vi "BonOMM-SAOMM.Test.vi"() -> ()   [LabVIEW 2011] (continued)
          n234 = property on="Offset OK" class="Bool (strict)"("DisabledEnum"=w454) -> ()  [unwired: 2 in, 2 out]
          n235 = local write "PixScale1"(w356) -> ()
          n236 = To Unsigned Word Integer(number=w325) -> (unsigned 16bit integer=w327:u16)
          n237 = To Unsigned Word Integer(number=w324) -> (unsigned 16bit integer=w326:u16)
          n238 = call-poly <vilib>:"Read Key.vi"("section"=w260, "error in (no error)"=w372, "key"="pixscale2", "refnum"=w367) -> ("error out"=w363:errorcluster, "value"=w355:dbl, "refnum out"=w364:T24)  [unwired: 4 in, 1 out]
          n239 = local write "Naxis2"(w327) -> ()
          n240 = local write "Naxis1"(w326) -> ()
          n241 = local write "PixScale2"(w355) -> ()
          n242 = property on="TableXYPos" class="XYGraph (strict)"("Active Cursor"=u32 0) -> (error out=w523:errorcluster)  [unwired: 2 in, 1 out]
          n243 = call-poly <vilib>:"Read Key.vi"("section"=w260, "error in (no error)"=w363, "key"="ROIWidth", "refnum"=w364) -> ("error out"=w365:errorcluster, "value"=w321:u32, "refnum out"=w366:T24)  [unwired: 4 in, 1 out]
          n244 = property on="TableXYPos" class="XYGraph (strict)"("PlotImages.Back"=picture data[5B] ("Plot Images:Back")) -> ()  [unwired: 2 in, 2 out]
          n245 = call-poly <vilib>:"Read Key.vi"("section"=w260, "error in (no error)"=w365, "key"="ROIHeight", "refnum"=w366) -> ("error out"=w273:errorcluster, "value"=w322:u32, "refnum out"=w274:T24)  [unwired: 4 in, 1 out]
          n246 = property on="ImgArray" class="IntGraph (strict)"("X Scale.Scale Fit"=w531, "Y Scale.Scale Fit"=w531, "Z Scale.Scale Fit"=u8 2) -> ()  [unwired: 2 in, 2 out]
          n247 = property on="LVDT-RA-coarse" class="WFGraph (strict)"("YScale.Maximum"=20.0 ("Y Scale.Range:Maximum"), "YScale.Minimum"=-3.0 ("Y Scale.Range:Minimum")) -> ()  [unwired: 2 in, 2 out]
          n248 = property on="TableXYPos" class="XYGraph (strict)"(error in=w523, "Cursor.Cursor X"=w519, "Cursor.Cursor Y"=w519) -> (error out=w524:errorcluster)  [unwired: 1 in, 1 out]
          n249 = property on="LowSNR" class="Bool (strict)"("Visible"=w215, "Blinking"=w215) -> ()  [unwired: 2 in, 2 out]
          n250 = property on="Saturé" class="Bool (strict)"("Visible"=w215, "Blinking"=w215) -> ()  [unwired: 2 in, 2 out]
          n251 = call-poly <vilib>:"Read Key.vi"("section"=w260, "error in (no error)"=w273, "key"="DefaultROIOffset", "refnum"=w274) -> ("error out"=w265:errorcluster, "value"=w266:u32, "refnum out"=w264:T24)  [unwired: 4 in, 1 out]
          n252 = To Unsigned Word Integer(number=w322) -> (unsigned 16bit integer=w323:u16)
          n253 = To Unsigned Word Integer(number=w321) -> (unsigned 16bit integer=w320:u16)
          n254 = local write "ROIHeight"(w323) -> ()
          n255 = local write "ROIWidth"(w320) -> ()
          n256 = property on="TableXYPos" class="XYGraph (strict)"(error in=w524, "Active Cursor"=u32 1) -> (error out=w522:errorcluster)  [unwired: 1 in, 1 out]
          n257 = call-poly <vilib>:"Read Key.vi"("section"=w260, "error in (no error)"=w265, "key"="DefaultBinning", "refnum"=w264) -> ("error out"=w254:errorcluster, "value"=w267:u32, "refnum out"=w255:T24)  [unwired: 4 in, 1 out]
          n258 = call-poly <vilib>:"Read Key.vi"("section"=w249, "error in (no error)"=w254, "key"="GuideRateRA", "refnum"=w255) -> ("error out"=w340:errorcluster, "value"=w331:dbl, "refnum out"=w341:T24)  [unwired: 4 in, 1 out]
          n259 = local write "RateRA"(w331) -> ()
          n260 = call-poly <vilib>:"Read Key.vi"("section"=w249, "error in (no error)"=w340, "key"="GuideRateDEC", "refnum"=w341) -> ("error out"=w247:errorcluster, "value"=w330:dbl, "refnum out"=w248:T24)  [unwired: 4 in, 1 out]
          n261 = local write "RateDEC"(w330) -> ()
          n262 = call-poly <vilib>:"Read Key.vi"("section"=w249, "error in (no error)"=w247, "key"="HexXRate", "refnum"=w248) -> ("error out"=w253:errorcluster, "value"=w244:dbl, "refnum out"=w252:T24)  [unwired: 4 in, 1 out]
          n263 = local write "HexXRate"(w244) -> ()
          n264 = call-poly <vilib>:"Read Key.vi"("section"=w249, "error in (no error)"=w253, "key"="HexYRate", "refnum"=w252) -> ("error out"=w245:errorcluster, "value"=w243:dbl, "refnum out"=w246:T24)  [unwired: 4 in, 1 out]
          n265 = local write "HexYRate"(w243) -> ()
          n266 = call-poly <vilib>:"Read Key.vi"("section"=w249, "error in (no error)"=w245, "key"="BacklashRA", "refnum"=w246) -> ("error out"=w339:errorcluster, "value"=w329:dbl, "refnum out"=w342:T24)  [unwired: 4 in, 1 out]
          n267 = local write "BacklashRA"(w329) -> ()
          n268 = call-poly <vilib>:"Read Key.vi"("section"=w249, "error in (no error)"=w339, "key"="BacklashDEC", "refnum"=w342) -> ("error out"=w346:errorcluster, "value"=w328:dbl, "refnum out"=w345:T24)  [unwired: 4 in, 1 out]
          n269 = local write "BacklashDEC"(w328) -> ()
          n270 = call-poly <vilib>:"Read Key.vi"("section"=w249, "error in (no error)"=w346, "key"="GuiderAgg", "refnum"=w345) -> ("error out"=w344:errorcluster, "value"=w332:dbl, "refnum out"=w343:T24)  [unwired: 4 in, 1 out]
          n271 = local write "Corr%"(w332) -> ()
          n272 = call-poly <vilib>:"Read Key.vi"("section"=w249, "error in (no error)"=w344, "key"="GuiderTreshold", "refnum"=w343) -> ("error out"=w335:errorcluster, "value"=w333:dbl, "refnum out"=w336:T24)  [unwired: 4 in, 1 out]
          n273 = local write "CorrTreshold"(w333) -> ()
          n274 = call-poly <vilib>:"Read Key.vi"("section"=w249, "error in (no error)"=w335, "key"="SNRTreshold", "refnum"=w336) -> ("error out"=w256:errorcluster, "value"=→"SNRtreshold":dbl, "refnum out"=w257:T24)  [unwired: 4 in, 1 out]
          n275 = call-poly <vilib>:"Read Key.vi"("section"=w258, "error in (no error)"=w256, "key"="UAxisOffset", "refnum"=w257) -> ("error out"=w281:errorcluster, "value"=w276:dbl, "refnum out"=w282:T24)  [unwired: 4 in, 1 out]
          n276 = local write "DefaultUAxisOffset"(w276) -> ()
          n277 = call-poly <vilib>:"Read Key.vi"("section"=w258, "error in (no error)"=w281, "key"="VAxisOffset", "refnum"=w282) -> ("error out"=w279:errorcluster, "value"=w275:dbl, "refnum out"=w280:T24)  [unwired: 4 in, 1 out]
          n278 = local write "DefaultVAxisOffset"(w275) -> ()
          n279 = call-poly <vilib>:"Read Key.vi"("section"=w258, "error in (no error)"=w279, "key"="Sampling", "refnum"=w280) -> ("error out"=w316:errorcluster, "value"=→"Sampling rate":i32, "refnum out"=w317:T24)  [unwired: 4 in, 1 out]
          n280 = call-poly <vilib>:"Read Key.vi"("section"=w258, "error in (no error)"=w316, "key"="DataLenght", "refnum"=w317) -> ("error out"=w238:errorcluster, "value"=w334:i32, "refnum out"=w237:T24)  [unwired: 4 in, 1 out]
          n281 = local write "ConsideredLenght"(w334) -> ()
          n282 = local write "Flat"(w473) -> ()
          n283 = call-poly <vilib>:"Read Key.vi"("section"=w207, "error in (no error)"=w238, "key"="PRAMMS-SG", "refnum"=w237) -> ("error out"=w213:errorcluster, "value"=w235:u32, "refnum out"=w214:T24)  [unwired: 4 in, 1 out]
          n284 = property on="TableXYPos" class="XYGraph (strict)"(error in=w522, "Cursor.Cursor X"=w518, "Cursor.Cursor Y"=w518) -> ()  [unwired: 1 in, 2 out]
          n285 = local write "Néon"(w473) -> ()
          n286 = local write "Signature"(w235) -> ()
          n287 = To Unsigned Word Integer(number=w267) -> (unsigned 16bit integer=w268:u16)
          n288 = To Unsigned Word Integer(number=w266) -> (unsigned 16bit integer=w270:u16)
          n289 = To Unsigned Word Integer(number=w266) -> (unsigned 16bit integer=w269:u16)
          n290 = local write "Arc"(w473) -> ()
          n291 = local write "Binning"(w268) -> ()
          n292 = local write "ROIYOffset"(w270) -> ()
          n293 = local write "ROIXOffset"(w269) -> ()
          n294 = local write "NeonOn"(w473) -> ()
          n295 = local write "ArcOn"(w473) -> ()
          n296 = global read "Globals.vi" "BonOMM VI Refnum"() -> (w283:refnum<vi>)
          n297 = call-poly <vilib>:"Read Key.vi"("section"=w207, "error in (no error)"=w213, "key"="tempspd", "refnum"=w214) -> ("error out"=w210:errorcluster, "value"=w204:u32, "refnum out"=w211:T24)  [unwired: 4 in, 1 out]
          n298 = local write "FlatOn"(w473) -> ()
          n299 = Initialize Array(0.0, 0) -> (w241:dbl[])
          n300 = Initialize Array(sgl 0.0, w516, w516) -> (w515:sgl[][])
          n301 = Bundle(w413, w413, w413) -> (w412:cluster{string, string, string})  [unwired: 1 in]
          n302 = local write "ImgData"(w515) -> ()
          n303 = local write "MC_connect"(FALSE) -> ()
          n304 = call-poly <vilib>:"Read Key.vi"("section"=w207, "error in (no error)"=w210, "key"="tempvrn", "refnum"=w211) -> ("error out"=w208:errorcluster, "value"=w205:string, "refnum out"=w209:T24)  [unwired: 4 in, 1 out]
          n305 = call-poly <vilib>:"Read Key.vi"("section"=w302, "error in (no error)"=w208, "key"="xgain", "refnum"=w209) -> ("error out"=w309:errorcluster, "value"=→"Gain X":dbl, "refnum out"=w308:T24)  [unwired: 4 in, 1 out]
          n306 = call-poly <vilib>:"Read Key.vi"("section"=w302, "error in (no error)"=w309, "key"="ygain", "refnum"=w308) -> ("error out"=w304:errorcluster, "value"=→"Gain Y":dbl, "refnum out"=w305:T24)  [unwired: 4 in, 1 out]
          n307 = call-poly <vilib>:"Read Key.vi"("section"=w302, "error in (no error)"=w304, "key"="zgain", "refnum"=w305) -> ("error out"=w314:errorcluster, "value"=→"Gain Z":dbl, "refnum out"=w313:T24)  [unwired: 4 in, 1 out]
          n308 = call-poly <vilib>:"Read Key.vi"("section"=w302, "error in (no error)"=w314, "key"="ugain", "refnum"=w313) -> ("error out"=w312:errorcluster, "value"=→"Gain U":dbl, "refnum out"=w311:T24)  [unwired: 4 in, 1 out]
          n309 = call-poly <vilib>:"Read Key.vi"("section"=w302, "error in (no error)"=w312, "key"="vgain", "refnum"=w311) -> ("error out"=w262:errorcluster, "value"=→"Gain V":dbl, "refnum out"=w263:T24)  [unwired: 4 in, 1 out]
          n310 = call-poly <vilib>:"Read Key.vi"("section"="options", "error in (no error)"=w262, "default value"=FALSE, "key"="autoconnect", "refnum"=w263) -> ("error out"=w378:errorcluster, "value"=w374:bool, "refnum out"=w379:T24)  [unwired: 3 in, 1 out]
          n311 = local write "AutoConnect?"(w374) -> ()
          n312 = call-poly <vilib>:"Read Key.vi"("section"=w382, "error in (no error)"=w378, "key"="secperpulse", "refnum"=w379) -> ("error out"=w392:errorcluster, "value"=w231:dbl, "refnum out"=w394:T24)  [unwired: 4 in, 1 out]
          "arcsec/pulse" <- w231
          n313 = call-poly <vilib>:"Read Key.vi"("section"=w382, "error in (no error)"=w392, "key"="naxis1", "refnum"=w394) -> ("error out"=w391:errorcluster, "value"=w232:dbl, "refnum out"=w393:T24)  [unwired: 4 in, 1 out]
          n314 = local write "NaxisMax"(w232) -> ()
          n315 = Multiply(x=w232, y=w231) -> (x*y=w230:dbl)
          n316 = call-poly <vilib>:"Read Key.vi"("section"=w382, "error in (no error)"=w391, "key"="represent", "refnum"=w393) -> ("error out"=w423:errorcluster, "value"=w420:dbl, "refnum out"=w424:T24)  [unwired: 4 in, 1 out]
          "Représentation" <- w420
          n317 = expression code="x/60"(w230) -> (→"RangeTable":dbl)
          n318 = call-poly <vilib>:"Read Key.vi"("section"=w382, "error in (no error)"=w423, "key"="cenx", "refnum"=w424) -> ("error out"=w505:errorcluster, "value"=w504:i32, "refnum out"=w506:T24)  [unwired: 4 in, 1 out]
          n319 = local write "CentreTel X"(w504) -> ()
          n320 = call-poly <vilib>:"Read Key.vi"("section"=w382, "error in (no error)"=w505, "key"="ceny", "refnum"=w506) -> ("error out"=w497:errorcluster, "value"=w503:i32, "refnum out"=w498:T24)  [unwired: 4 in, 1 out]
          n321 = local write "CentreTel Y"(w503) -> ()
          n322 = call-poly <vilib>:"Read Key.vi"("section"=w382, "error in (no error)"=w497, "key"="refx", "refnum"=w498) -> ("error out"=w502:errorcluster, "value"=w496:i32, "refnum out"=w501:T24)  [unwired: 4 in, 1 out]
          n323 = local write "Reference X"(w496) -> ()
          n324 = call-poly <vilib>:"Read Key.vi"("section"=w382, "error in (no error)"=w502, "key"="refy", "refnum"=w501) -> ("error out"=w433:errorcluster, "value"=w495:i32, "refnum out"=w434:T24)  [unwired: 4 in, 1 out]
          n325 = local write "Reference Y"(w495) -> ()
          n326 = Less Or Equal?(x=w420, y=70.0) -> (x <= y?=w418:bool)
          n327 = call-poly <vilib>:"Read Key.vi"("section"=w382, "error in (no error)"=w433, "key"="rangex", "refnum"=w434) -> ("error out"=w435:errorcluster, "value"=w438:i32, "refnum out"=w436:T24)  [unwired: 4 in, 1 out]
          n328 = local write "Rangement X"(w438) -> ()
          n329 = Select(t=T17."Enabled" ("Disabled"), s=w418, f=T17."Disabled" ("Disabled")) -> (s? t:f=w415:T17)
          n330 = call-poly <vilib>:"Read Key.vi"("section"=w382, "error in (no error)"=w435, "key"="rangey", "refnum"=w436) -> ("error out"=w429:errorcluster, "value"=w439:i32, "refnum out"=w430:T24)  [unwired: 4 in, 1 out]
          n331 = local write "Rangement Y"(w439) -> ()
          n332 = property on="GetDSS" class="Bool (strict)"("DisabledEnum"=w415) -> ()  [unwired: 2 in, 2 out]
          n333 = call-poly <vilib>:"Read Key.vi"("section"=w382, "error in (no error)"=w429, "key"="rangez", "refnum"=w430) -> ("error out"=w427:errorcluster, "value"=w426:i32, "refnum out"=w428:T24)  [unwired: 4 in, 1 out]
          n334 = local write "Rangement Z"(w426) -> ()
          n335 = call-poly <vilib>:"Read Key.vi"("section"=w382, "error in (no error)"=w427, "key"="vrapid", "refnum"=w428) -> ("error out"=w465:errorcluster, "value"=→"vitesse rapide":dbl, "refnum out"=w464:T24)  [unwired: 4 in, 1 out]
          n336 = call-poly <vilib>:"Read Key.vi"("section"=w382, "error in (no error)"=w465, "key"="vlente", "refnum"=w464) -> ("error out"=w471:errorcluster, "value"=→"vitesse lente":dbl, "refnum out"=w470:T24)  [unwired: 4 in, 1 out]
          n337 = call-poly <vilib>:"Read Key.vi"("section"=w382, "error in (no error)"=w471, "key"="accel", "refnum"=w470) -> ("error out"=w466:errorcluster, "value"=→"accelleration":dbl, "refnum out"=w467:T24)  [unwired: 4 in, 1 out]
          n338 = call-poly <vilib>:"Read Key.vi"("section"=w382, "error in (no error)"=w466, "key"="vfocus", "refnum"=w467) -> ("error out"=w385:errorcluster, "value"=→"vitesse focus":dbl, "refnum out"=w386:T24)  [unwired: 4 in, 1 out]
          n339 = call-poly <vilib>:"Read Key.vi"("section"=w382, "error in (no error)"=w385, "key"="vjog", "refnum"=w386) -> ("error out"=w383:errorcluster, "value"=→"vitesse jog":dbl, "refnum out"=w384:T24)  [unwired: 4 in, 1 out]
          n340 = call <vilib>:"Close Config Data.vi"("error in (no error)"=w383, "refnum"=w384) -> ("file path"=w443:path)  [unwired: 8 in, 1 out]
          n341 = call "Readwindowpropfile.vi"("configuration file path"=w443) -> ("PanelOrigin"=w285:cluster{"panelx":i16, "panely":i16}, "MinimumSize"=w286:cluster{"Horizontal":i16, "Vertical":i16}, "PanelBounds"=w287:T25, "resizable"=w288:bool, "AllFound"=w284:bool)  [unwired: 6 in]
          n342 = Bundle(w241, w241) -> (w449:cluster{dbl[], dbl[]})  [unwired: 1 in]
          n343 = Initialize Array(w412, 0) -> (→"CmdDone":cluster{string, string, string}[])
          n344 = flat-sequence {
            tunnel: w283 -> [w558]
            tunnel: w288 -> [w559]
            tunnel: w287 -> [w560]
            tunnel: w286 -> [w554]
            tunnel: [w561] -> w295
            tunnel: w285 -> [w561]
            tunnel: [w557] -> w294
            tunnel: [w560] -> w293
            tunnel: [w559] -> w292
            tunnel: [w555] -> w291
            tunnel: [w554] -> w290
            tunnel: w295 -> [w567]
            tunnel: [w567] -> w289
            tunnel: w294 -> [w566]
            tunnel: w293 -> [w565]
            tunnel: w292 -> [_]
            tunnel: w291 -> [w564]
            tunnel: w290 -> [w563]
            tunnel: w289 -> [w573]
            frame #0 {
              n345 = property class="VI"(reference=w558, "Front Panel.Resizeable"=TRUE ("Front Panel Window:Resizable")) -> (reference out=w557:refnum<vi>, error out=w555:errorcluster)  [unwired: 1 in]
            }
            frame #1 {
              n346 = disable-structure shown="Disabled" {
                disable-tunnel: w566 -> [w572 _]
                disable-tunnel: w565 -> [w571 _]
                disable-tunnel: w564 -> [w570 _]
                disable-tunnel: w563 -> [w569 _]
                disable-tunnel: TRUE ("Front Panel Window:Resizable") -> [w568 _]
                frame Disabled {
                  n347 = property class="VI"(reference=w572, error in=w570, "Front Panel.Resizeable"=w568, "Front Panel.PanelBounds"=w571, "Minimum Panel Size"=w569) -> ()  [unwired: 2 out]
                }
                frame Enabled {
                }
              }
            }
            frame #2 {
              n348 = property on="Pane" class="Pane"("Origin"=w573) -> ()  [unwired: 2 in, 2 out]
              n349 = property on="MainTab" class="TabCtl (strict)"("Position"=cluster{i32, i32} {0, 0}) -> ()  [unwired: 2 in, 2 out]
            }
            frame #3 {
              "Lecture Configuration" <- TRUE ("Lecture Configuration")
            }
          }
          n350 = case shown="True" w284 {
            frame False {
              # "Ne devrais pas arriver ..."
              n351 = One Button Dialog(message="Impossible de trouver le fichier properties.ini\nUtilisation des valeurs par défauts ...") -> ()  [unwired: 1 in, 1 out]
            }
            frame True {
            }
          }
          n352 = local write "LVDT-RA-Data"(w241) -> ()
          n353 = call "Draw_crosshair.vi"("Image IN"=w515, "White Value"=sgl 255.0) -> ("Image OUT"=w514:sgl[][])  [unwired: 13 in]
          n354 = Initialize Array(w449, 0) -> (w242:cluster{dbl[], dbl[]}[])
          n355 = Initialize Array("", 0) -> (w458:string[])
          n356 = Initialize Array(refnum<k5> refnum ("External TCP ID 2"), 0) -> (w456:refnum<k5>[])
          n357 = local write "subimg"(w514) -> ()
          n358 = local write "Img DEC"(w425) -> ()
          n359 = local write "RA-USNO"(w425) -> ()
          n360 = local write "DEC-USNO"(w425) -> ()
          n361 = local write "Img RA"(w425) -> ()
          n362 = local write "Graph-Flux"(w242) -> ()
          n363 = local write "Graph-Centroids"(w242) -> ()
          n364 = local write "Graph-SNR"(w242) -> ()
          n365 = local write "ImageUsage"(w373) -> ()
          n366 = disable-structure shown="Enabled" {
            disable-tunnel: w205 -> [w552 _]
            disable-tunnel: w204 -> [w551 _]
            frame Disabled {
              n367 = Type Cast(type=refnum<visa-resource-name> "-1" ("Table VRN"), x=w552) -> (*(type *) &x=w546:refnum<visa-resource-name>)
              n368 = local write "HexTemp Baud rate"(w551) -> ()
              n369 = local write "HexTemp VRN"(w546) -> ()
              n370 = call-poly "VISA Configure Serial Port"("VISA resource name"=w546, "timeout (10sec)"=u32 1000, "Enable Termination\nChar (T)"=FALSE ("Enable Termination\nChar (T)"), "baud rate (9600)"=w551) -> ("error out"=w547:errorcluster)  [unwired: 10 in, 1 out]
              n371 = local write "HexapodeTempError"(w547) -> ()
            }
            frame Enabled {
            }
          }
          n372 = local write "Clients ID"(w456) -> ()
          n373 = local write "Clients"(w458) -> ()
          n374 = local write "Hex-XGraph"(w242) -> ()
          n375 = local write "Guiderreur"(w242) -> ()
          n376 = local write "Hex-YGraph"(w242) -> ()
          n377 = local write "Cumulatif"(w242) -> ()
          n378 = local write "CumulativeError"(w242) -> ()
          n379 = local write "CentroidsData"(w242) -> ()
          n380 = local write "HexXData"(w242) -> ()
          n381 = local write "HexYData"(w242) -> ()
          n382 = local write "SNRData"(w242) -> ()
          n383 = local write "FluxData"(w242) -> ()
          "RAtmp" <- w425
          "Dectmp" <- w425
          "Menu Error" <- w461
          "VI Reference Error" <- w461
          "Starry Night Error" <- w461
          "Excom Error" <- w461
          "Guider Error" <- w461
          "ActiveX Error" <- w461
          "Critical Error" <- w461
          "Config Error" <- w461
          "Serial Error" <- w461
          "TCP/IP Error" <- w461
          "wget error" <- w461
          "TCS Error" <- w461
          "File I/O Error" <- w461
          "FIFO actif" <- w233
          "TCS actif" <- w233
          "TCS C actif" <- w233
          "Table actif" <- w233
          "Integrating" <- w233
          "MovingXY" <- w233
          "MovingZ" <- w233
          "CorrectZ" <- w233
          "CorrectXY" <- w233
          "Focusing" <- w233
          "CurvCorrect" <- w233
          "SubIMG4DSS?" <- w233
        }
      }
      n384 = property on="Déc étoile guide" class="DigNum (strict)"("Visible"=w200) -> ()  [unwired: 2 in, 2 out]
      n385 = property on="A.D. étoile guide" class="DigNum (strict)"("Visible"=w200) -> ()  [unwired: 2 in, 2 out]
      n386 = property on="Graph-Centroids" class="XYGraph (strict)"("Visible"=w200) -> ()  [unwired: 2 in, 2 out]
      n387 = property on="Flux Max" class="DigNum (strict)"("Visible"=w200) -> ()  [unwired: 2 in, 2 out]
      n388 = property on="Guiderreur" class="XYGraph (strict)"("Visible"=w200) -> ()  [unwired: 2 in, 2 out]
      n389 = property on="Flux inst." class="DigNum (strict)"("Visible"=w200) -> ()  [unwired: 2 in, 2 out]
      n390 = property on="StopCam" class="Bool (strict)"("Visible"=w200) -> ()  [unwired: 2 in, 2 out]
      n391 = property on="GoCam" class="Bool (strict)"("Visible"=w200) -> ()  [unwired: 2 in, 2 out]
      n392 = property on="Approaching limit" class="Bool (strict)"("Visible"=w202, "Blinking"=w202) -> ()  [unwired: 2 in, 2 out]
      n393 = property on="Target OutofRange" class="Bool (strict)"("Visible"=w202, "Blinking"=w202) -> ()  [unwired: 2 in, 2 out]
      n394 = property on="Lampe Allumée ?" class="Bool (strict)"("Visible"=w202, "Blinking"=w202) -> ()  [unwired: 2 in, 2 out]
      n395 = property on="ModeInv" class="Bool (strict)"("Visible"=w202, "Blinking"=w202) -> ()  [unwired: 2 in, 2 out]
      n396 = property on="StarFaded?" class="Bool (strict)"("Visible"=w202, "Blinking"=w202) -> ()  [unwired: 2 in, 2 out]
      n397 = property on="Alarme PRAMS" class="Bool (strict)"("Visible"=w202, "Blinking"=w202) -> ()  [unwired: 2 in, 2 out]
      n398 = property on="Picture" class="Pict"("Visible"=w201) -> ()  [unwired: 2 in, 2 out]
      n399 = property on="filtre_nom" class="Str"("Visible"=w201) -> ()  [unwired: 2 in, 2 out]
      n400 = property on="q-raf" class="Bool (strict)"("Visible"=w201) -> ()  [unwired: 2 in, 2 out]
      n401 = property on="cancel-raf" class="Bool (strict)"("Visible"=w201) -> ()  [unwired: 2 in, 2 out]
      n402 = property on="change_filtre_liste" class="Bool (strict)"("Visible"=w201) -> ()  [unwired: 2 in, 2 out]
      n403 = property on="ChoixFiltre" class="Clust (strict)"("Visible"=w201) -> ()  [unwired: 2 in, 2 out]
      n404 = property on="F#" class="DigNum (strict)"("Visible"=w201) -> ()  [unwired: 2 in, 2 out]
      n405 = property on="ST-" class="Bool (strict)"("Visible"=w201) -> ()  [unwired: 2 in, 2 out]
      n406 = property on="ST+" class="Bool (strict)"("Visible"=w201) -> ()  [unwired: 2 in, 2 out]
      n407 = property on="SET ZERO" class="Bool"("Visible"=w201) -> ()  [unwired: 2 in, 2 out]
      n408 = property on="ST_RAZ" class="Bool"("Visible"=w201) -> ()  [unwired: 2 in, 2 out]
      n409 = property on="reconnect" class="Bool (strict)"("Visible"=w201) -> ()  [unwired: 2 in, 2 out]
      n410 = property on="ST_SPD" class="Slide (strict)"("Visible"=w201) -> ()  [unwired: 2 in, 2 out]
    }
    frame #4 {
      # "Initialisation des éléments du menu"
      n411 = case shown="True" w576 {
        frame False {
        }
        frame True {
          w649 = refnum<visa-resource-name> "-1" ("Table VRN")
          # "Désactive les filtres"
          # "Menu \"Roue à filtre\""
          # "Menu \"Tables de guidage\""
          # "Menu \"Caméra de référence\""
          # "Menu \"Secondaire Actif\""
          # "Menu \"Télescope\""
          # "Menu des scripts"
          # "Menu des Instruments"
          # "Menu des communications"
          # "Ajoute les items de menu custom"
          # "Enlève les items de menu non-utilisés"
          n412 = Current VI's Menubar ("Barre de menu")() -> (w693:refnum<k9>)
          n413 = Delete Menu Items(7:string[] ["APP_EDIT", "APP_VIEW", "APP_PROJECT", "APP_TOOLS"], 9:w693) -> (0:w651:errorcluster, 3:w652:refnum<k9>)  [unwired: 2 in]
          n414 = call "MenuFixer.vi"("Menu Name"=string[] ["Communications", "Instruments", "Scripts et Automatismes", "Télescope", "Secondaire Actif", "Caméra de référence", "Tables de guidage", "Roue à filtres"] ("Array Constant"), "Prefix"="main_") -> ("Item Tags"=w592:string[], "Item Names"=w591:string[])  [unwired: 8 in]
          n415 = call "MenuFixer.vi"("Menu Name"=string[] ["Charger la librairie de la queue", "Charger une librairie d'objets", "APP_SEPARATOR", "Déterminer l'astrométrie du champ", "Calibration du foyer automatique", "APP_SEPARATOR", "Construction d'une LUT"] ("menuelem_cmd"), "Prefix"="scp_") -> ("Item Tags"=w604:string[], "Item Names"=w603:string[])  [unwired: 8 in]
          n416 = Insert Menu Items(4:"APP_OPERATE" ("after item"), 6:w651, 7:w592, 8:w591, 9:w652) -> (0:w642:errorcluster, 3:w643:refnum<k9>)  [unwired: 1 in, 1 out]
          n417 = call "MenuFixer.vi"("Menu Name"=string[] ["Telescope Control System", "Caméra de référence", "Tables de guidage", "Secondaire Actif", "Module de calibration", "MC-BonOMM", "Commandes externes", "Station Météo", "APP_SEPARATOR", "Reconnexion automatique ?"] ("menu_comm"), "Prefix"="com_") -> ("Item Tags"=w590:string[], "Item Names"=w596:string[])  [unwired: 8 in]
          n418 = Insert Menu Items(5:"main_Communications" ("menu tag"), 6:w642, 7:w590, 8:w596, 9:w643) -> (0:w685:errorcluster, 3:w686:refnum<k9>)  [unwired: 1 in, 1 out]
          n419 = call "MenuFixer.vi"("Menu Name"=string[] ["Synchroniser la coupole", "Synchroniser les horloges", "Modifier la vitesse du télescope", "Modifier la vitesse de guidage", "Modifier l'époque d'affichage", "APP_SEPARATOR", "Reconnexion"] ("menuelem_cmd"), "Prefix"="tel_") -> ("Item Tags"=w609:string[], "Item Names"=w608:string[])  [unwired: 8 in]
          n420 = Index Array(array=w590) -> (element #1=w676:string, element #2=w675:string, element #3=w674:string, element #4=w644:string, element #5=w657:string, element #6=w656:string, element #7=w655:string, element #8=w654:string, element #10=w653:string)  [unwired: 10 in, 1 out]
          n421 = local read "TCS VRN"() -> (w682:refnum<visa-resource-name>)
          n422 = Not Equal?(x=w682, y=w649) -> (x != y?=w667:bool)
          n423 = local write "TCS COMM"(w667) -> ()
          n424 = Set Menu Item Info(6:w667, 7:w676, 8:w685, 11:w686) -> (0:w688:errorcluster, 3:w687:refnum<k9>)  [unwired: 3 in]
          n425 = local read "PrAMS VRN"() -> (w681:refnum<visa-resource-name>)
          n426 = Not Equal?(x=w681, y=w649) -> (x != y?=w666:bool)
          n427 = local write "PrAMS COMM"(w666) -> ()
          n428 = Set Menu Item Info(6:w666, 7:w675, 8:w688, 11:w687) -> (0:w690:errorcluster, 3:w689:refnum<k9>)  [unwired: 3 in]
          n429 = local read "Table VRN"() -> (w680:refnum<visa-resource-name>)
          n430 = call "MenuFixer.vi"("Menu Name"=string[] ["Paramètres d'asservissement", "Commander l'hexapode", "Panneau de offset", "Déplacement manuel", "APP_SEPARATOR", "Remise à zéro", "APP_SEPARATOR", "Reconnexion"] ("menuelem_cmd"), "Prefix"="hex_") -> ("Item Tags"=w613:string[], "Item Names"=w612:string[])  [unwired: 8 in]
          n431 = Not Equal?(x=w680, y=w649) -> (x != y?=w665:bool)
          n432 = local write "TableCOM"(w665) -> ()
          n433 = Set Menu Item Info(6:w665, 7:w674, 8:w690, 11:w689) -> (0:w645:errorcluster, 3:w648:refnum<k9>)  [unwired: 3 in]
          n434 = local read "Hexapod VRN"() -> (w650:refnum<visa-resource-name>)
          n435 = Not Equal?(x=w650, y=w649) -> (x != y?=w623:bool)
          n436 = local write "Hexapod COMM"(w623) -> ()
          n437 = Set Menu Item Info(6:w623, 7:w644, 8:w645, 11:w648) -> (0:w646:errorcluster, 3:w647:refnum<k9>)  [unwired: 3 in]
          n438 = local read "Calib VRN"() -> (w679:refnum<visa-resource-name>)
          n439 = Not Equal?(x=w679, y=w649) -> (x != y?=w662:bool)
          n440 = local write "Calib COMM"(w662) -> ()
          n441 = Set Menu Item Info(6:w662, 7:w657, 8:w646, 11:w647) -> (0:w692:errorcluster, 3:w691:refnum<k9>)  [unwired: 3 in]
          n442 = local read "MC-BonOMM VRN"() -> (w678:refnum<visa-resource-name>)
          n443 = call "MenuFixer.vi"("Menu Name"=string[] ["Enregistrer la prochaine image", "Modifier les paramètres", "Modifier la région d'intérêt", "APP_SEPARATOR", "Binning 1x1", "Binning 2x2", "Binning 4x4", "Binning 5x5", "APP_SEPARATOR", "Reconnexion"] ("menuelem_cmd"), "Prefix"="cam_") -> ("Item Tags"=w618:string[], "Item Names"=w617:string[])  [unwired: 8 in]
          n444 = Not Equal?(x=w678, y=w649) -> (x != y?=w663:bool)
          n445 = local write "MCB COMM"(w663) -> ()
          n446 = Set Menu Item Info(6:w663, 7:w656, 8:w692, 11:w691) -> (0:w683:errorcluster, 3:w684:refnum<k9>)  [unwired: 3 in]
          n447 = local read "Excmd VRN"() -> (w677:refnum<visa-resource-name>)
          n448 = Not Equal?(x=w677, y=w649) -> (x != y?=w664:bool)
          n449 = Set Menu Item Info(6:w664, 7:w655, 8:w683, 11:w684) -> (0:w672:errorcluster, 3:w673:refnum<k9>)  [unwired: 3 in]
          n450 = local write "ExCmd COMM"(w664) -> ()
          n451 = local read "Cx"() -> (w671:bool)
          n452 = local read "AutoConnect?"() -> (w660:bool)
          n453 = Set Menu Item Info(6:w671, 7:w654, 8:w672, 11:w673) -> (0:w658:errorcluster, 3:w659:refnum<k9>)  [unwired: 3 in]
          n454 = call "MenuFixer.vi"("Menu Name"=string[] ["Modifier les vitesses des tables", "Positions prédéfinies", "Commandes XYZ", "APP_SEPARATOR", "Modifier les paramètres", "APP_SEPARATOR", "Reconnexion"] ("menuelem_cmd"), "Prefix"="tab_") -> ("Item Tags"=w622:string[], "Item Names"=w621:string[])  [unwired: 8 in]
          n455 = Set Menu Item Info(6:w660, 7:w653, 8:w658, 11:w659) -> (0:w661:errorcluster, 3:w599:refnum<k9>)  [unwired: 3 in]
          n456 = local read "instruments.ini"() -> (w668:path)
          n457 = local read "Tableau des filtres"() -> (w577:string[])
          n458 = call "RaFMenuFixer.vi"("Tableau des filtres"=w577, "Prefix"="raf_") -> ("Item Tags"=w578:string[], "Item Names"=w579:string[])  [unwired: 8 in]
          n459 = call <vilib>:"Open Config Data.vi"("create file if necessary (T)"=FALSE, "configuration file path"=w668) -> ("error out"=w699:errorcluster, "refnum"=w700:T24)  [unwired: 7 in, 1 out]
          n460 = Array Size(array=w577) -> (size(s)=w584:i32)
          n461 = call <vilib>:"Get Section Names.vi"("error in (no error)"=w699, "refnum"=w700) -> ("error out"=w694:errorcluster, "section names"=w669:string[], "refnum out"=w695:T24)  [unwired: 7 in]
          "section names" <- w669
          n462 = Array Subset(array=w578, index=2, length=w584) -> (w581:string[])
          n463 = Array Subset(array=w579, index=2, length=w584) -> (w580:string[])
          n464 = call <vilib>:"Close Config Data.vi"("error in (no error)"=w694, "refnum"=w695) -> ()  [unwired: 8 in, 2 out]
          n465 = Build Array (concatenate)(w669, "APP_SEPARATOR", "Modifier les paramètres") -> (w601:string[])
          n466 = call "MenuFixer.vi"("Menu Name"=w601, "Prefix"="ins_") -> ("Item Tags"=w600:string[], "Item Names"=w598:string[])  [unwired: 8 in]
          n467 = Insert Menu Items(5:"main_Instruments" ("menu tag"), 6:w661, 7:w600, 8:w598, 9:w599) -> (0:w636:errorcluster, 3:w637:refnum<k9>)  [unwired: 1 in, 1 out]
          n468 = Insert Menu Items(5:"main_Scripts et Automatismes" ("menu tag"), 6:w636, 7:w604, 8:w603, 9:w637) -> (0:w638:errorcluster, 3:w639:refnum<k9>)  [unwired: 1 in, 1 out]
          n469 = Insert Menu Items(5:"main_Télescope" ("menu tag"), 6:w638, 7:w609, 8:w608, 9:w639) -> (0:w633:errorcluster, 3:w634:refnum<k9>)  [unwired: 1 in, 1 out]
          n470 = Insert Menu Items(5:"main_Secondaire Actif" ("menu tag"), 6:w633, 7:w613, 8:w612, 9:w634) -> (0:w630:errorcluster, 3:w631:refnum<k9>)  [unwired: 1 in, 1 out]
          n471 = Insert Menu Items(5:"main_Caméra de référence" ("menu tag"), 6:w630, 7:w618, 8:w617, 9:w631) -> (0:w627:errorcluster, 3:w628:refnum<k9>)  [unwired: 1 in, 1 out]
          n472 = Insert Menu Items(5:"main_Tables de guidage " ("menu tag"), 6:w627, 7:w622, 8:w621, 9:w628) -> (0:w624:errorcluster, 3:w625:refnum<k9>)  [unwired: 1 in, 1 out]
          n473 = Insert Menu Items(5:"main_Roue à filtres" ("menu tag"), 6:w624, 7:w578, 8:w579, 9:w625) -> (0:w586:errorcluster, 3:w589:refnum<k9>)  [unwired: 1 in, 1 out]
          n474 = for {
            tunnel: [w708] -> w588
            tunnel: w589 -> [w710]
            tunnel: w586 -> [w709]
            tunnel: [w707] -> w587
            tunnel: w581 -> [w705] mode=indexing
            tunnel: w580 -> [w704] mode=indexing
            w706 = FALSE ("enabled")
            n475 = Set Menu Item Info(6:w706, 7:w705, 8:w709, 9:w706, 10:w704, 11:w710) -> (0:w707:errorcluster, 3:w708:refnum<k9>)  [unwired: 1 in]
          }
          n476 = flat-sequence {
            tunnel: w588 -> [w712]
            tunnel: w587 -> [w711]
            frame #0 {
              n477 = local write "Menu Error"(w711) -> ()
              "menu ref" <- w712
            }
            frame #1 {
              "Gestion des menus" <- TRUE ("Gestion des menus")
            }
          }
        }
      }
    }
    frame #5 {
      # "Initialisation de SAOMM"
      n478 = case shown="True" w714 {
        frame False {
        }
        frame True {
          n479 = flat-sequence {
            tunnel: [TRUE] -> w715
            frame #0 {
              w717 = 0 ("Signature")
              w720 = 0 ("Nb_ACK")
              w718 = FALSE ("PRAMMS actif")
              # "Mettre dans le fichier de configuration ..."
              # "Signature Sale ..."
              n480 = local read "path_config"() -> (w728:path)
              n481 = Build Path(base path=w728, name or relative path=path "command.ini" ("command.ini")) -> (appended path=w726:path)
              n482 = call "SAOMM-BuildTypeArray.vi"("command.ini"=w726) -> ("CommandArray"=→"MessageType":cluster{string[], u32[]})  [unwired: 14 in]
              n483 = local write "Signature"(u32 1886544237 ("Signature")) -> ()
              n484 = local write "PrAMS-ACK"(w717) -> ()
              n485 = local write "Hexapod-ACK"(w717) -> ()
              n486 = local write "LastProcSavedID"(u64 0 ("LastProcSavedID")) -> ()
              n487 = local read "properties.ini"() -> (w724:path)
              n488 = local write "Nb_ACK (PrAMS)"(w720) -> ()
              n489 = local write "Nb_ACK (hex)"(w720) -> ()
              n490 = local write "Nb_Error (PrAMS)"(w720) -> ()
              n491 = local write "Nb_Error (hex)"(w720) -> ()
              n492 = local write "ImgArray"(u32[][] [] ("ImgArray")) -> ()
              n493 = call "SAOMM-ROIEnums.vi"("Path"=w724) -> ("StringEnums"=w723:string[], "ROISizes"=→"ROISizes":i32[])  [unwired: 13 in]
              n494 = local write "CorrDelay"(u32 5000 ("CorrDelay")) -> ()
              n495 = local write "QueryingHexapod"(w718) -> ()
              n496 = local write "PrAMS-Error"(w718) -> ()
              n497 = local write "Servo"(w718) -> ()
              n498 = local write "HexaCons actif"(w718) -> ()
              n499 = local write "Hexapod-Error"(w718) -> ()
              n500 = local write "LastProcID"(u64 0 ("Last Received ID")) -> ()
              n501 = property on="ROIsurface" class="Ring (strict)"("Strings []"=w723) -> ()  [unwired: 2 in, 2 out]
              "PrAMS Error" <- errorcluster {"status"=FALSE, "code"=0, "source"=""} ("PRAMMS Error")
              "PrAMS actif" <- w718
              "HxMoving" <- w718
              "Exceptions" <- T19 {"Command Error"=FALSE, "Slip/Stall"=FALSE, "Overtravel"=FALSE, "Done"=FALSE, "nError"=0.0, "nSlip"=0.0, "nOT"=0.0, "nDone"=0.0} ("Newmark-Exceptions")
            }
            frame #1 {
              w734 = T17."Enabled" ("Disabled")
              w735 = T17."Disabled and Grayed Out" ("Disabled")
              w737 = u16 0 items=["Opération Fixe", "Asservissement Ouvert", "Asservissement Fermé", "Calibration"] ("Mode")
              w733 = u32 0 ("ListenerExec")
              w738 = u16 2 items=["1 x 1"=1, "2 x 2"=2, "4 x 4"=4, "5 x 5"=5] ("Binning")
              n502 = local write "GetOptimalTime"(w733) -> ()
              n503 = local write "GetOptimalTime"(w733) -> ()
              n504 = local write "Nb_FalconProc_demandé"(w733) -> ()
              n505 = local write "SetBinningTime"(w733) -> ()
              n506 = local write "Nb_FalconProc_reçu"(w733) -> ()
              n507 = local write "SetFPSTime"(w733) -> ()
              n508 = local write "SetROITime"(w733) -> ()
              n509 = local write "StopTime"(w733) -> ()
              n510 = local write "FalconQuery"(w733) -> ()
              n511 = local write "HexapodQuery"(w733) -> ()
              n512 = local write "ListenerExec"(w733) -> ()
              n513 = local write "SetExpTime"(w733) -> ()
              n514 = local write "StartTime"(w733) -> ()
              n515 = local write "Dump"("" ("Dump")) -> ()
              n516 = local write "Binning"(w738) -> ()
              n517 = local write "Mode"(w737) -> ()
              n518 = property on="GoCam" class="Bool (strict)"("DisabledEnum"=w734) -> ()  [unwired: 2 in, 2 out]
              n519 = property on="StopCam" class="Bool (strict)"("DisabledEnum"=w734) -> ()  [unwired: 2 in, 2 out]
              n520 = property on="XReference" class="DigNum (strict)"("DisabledEnum"=w734) -> ()  [unwired: 2 in, 2 out]
              n521 = property on="YReference" class="DigNum (strict)"("DisabledEnum"=w734) -> ()  [unwired: 2 in, 2 out]
              n522 = property on="Mode" class="Ring (strict)"("DisabledEnum"=w735) -> ()  [unwired: 2 in, 2 out]
              n523 = property on="StartServo" class="Bool (strict)"("DisabledEnum"=w735) -> ()  [unwired: 2 in, 2 out]
              n524 = property on="StopServo" class="Bool (strict)"("DisabledEnum"=w735) -> ()  [unwired: 2 in, 2 out]
            }
            frame #2 {
              w739 = -1.0 ("LastImageTime")
              # "Initialisation des tableaux de données ..."
              n525 = local read "properties.ini"() -> (w748:path)
              n526 = Initialize Array(-inf ("LastImageTime"), 5 ("dimension size")) -> (w763:dbl[])
              n527 = local read "path_config"() -> (w741:path)
              n528 = local write "FalconProcTimeStamp"(w739) -> ()
              n529 = local write "LastImageTime"(w739) -> ()
              n530 = local write "LastSaveTimeStamp"(w739) -> ()
              n531 = call <vilib>:"Open Config Data.vi"("create file if necessary (T)"=FALSE, "configuration file path"=w748) -> ("error out"=w746:errorcluster, "refnum"=w745:T24)  [unwired: 7 in, 1 out]
              n532 = local read "Signature"() -> (w761:u32)
              n533 = local write "H_LUT"(w763) -> ()
              n534 = local write "H_Offset"(w763) -> ()
              n535 = local write "H_Servo"(w763) -> ()
              n536 = local write "H_Console"(w763) -> ()
              n537 = local write "H_Position"(w763) -> ()
              n538 = Build Path(base path=w741, name or relative path=path "command.ini" ("command.ini")) -> (appended path=w740:path)
              n539 = call-poly <vilib>:"Read Key.vi"("section"="communications" ("key"), "error in (no error)"=w746, "key"="PRAMMS-IP", "refnum"=w745) -> ("error out"=w752:errorcluster, "value"=w744:string, "refnum out"=w751:T24)  [unwired: 4 in, 1 out]
              n540 = call "Hexapod-connect.vi"("IP"=w744, "Port"=u16 10010, "Signature"=w761, "path_config"=w740) -> ("connection ID"=w758:refnum<k5>, "Connexion"=→"Connexion":bool, "Lecture"=→"Lecture":bool, "Écriture"=→"Écriture":bool, "Error OUT"=w756:errorcluster)  [unwired: 7 in]
              n541 = call <vilib>:"Close Config Data.vi"("error in (no error)"=w752, "refnum"=w751) -> ()  [unwired: 8 in, 2 out]
              n542 = local read "Hexapod VRN"() -> (w760:refnum<visa-resource-name>)
              n543 = case shown="Error" w756 {
                frame No Error {
                }
                frame Error {
                  n544 = One Button Dialog(message="Erreur lors de la connexion\nà l'hexapode-console.") -> ()  [unwired: 1 in, 1 out]
                }
              }
              n545 = Type Cast(type=w744, x=w758) -> (*(type *) &x=w757:string)
              n546 = Type Cast(type=w760, x=w757) -> (*(type *) &x=w759:refnum<visa-resource-name>)
              n547 = local write "Hexapod VRN"(w759) -> ()
            }
          }
          "PrAMS + Hexapode" <- w715
        }
      }
    }
    frame #6 {
      # "Configure les paramètres par défaut de PrAMS et Hexapode-Console"
      n548 = case shown="True" w767 {
        frame False {
        }
        frame True {
          n549 = flat-sequence {
            frame #0 {
              w768 = u16 1 items=["Initialisation", "Retirer la lame séparatrice du faisceau", "Mettre la lame séparatrice dans le faisceau"] ("SpliterSelector")
              n550 = local write "SpliterSelector"(w768) -> ()
            }
            frame #1 {
              n551 = local read "path_config"() -> (w771:path)
              n552 = local read "PrAMS VRN"() -> (w780:refnum<visa-resource-name>)
              n553 = local read "Binning"() -> (w775:u16)
              n554 = local read "PrAMS Error"() -> (w778:errorcluster)
              n555 = local read "Signature"() -> (w779:u32)
              n556 = local read "ROIWidth"() -> (w774:u16)
              n557 = local read "ROIHeight"() -> (w773:u16)
              n558 = local read "ROIXOffset"() -> (w776:u16)
              n559 = local read "ROIYOffset"() -> (w777:u16)
              n560 = Build Path(base path=w771, name or relative path=path "command.ini" ("command.ini")) -> (appended path=w769:path)
              n561 = call "SAOMM-FalconFixer_patched.vi"("PRAMMS VRN"=w780, "ROIYOffset"=w777, "ROIXOffset"=w776, "Binning"=w775, "command.ini"=w769, "Signature"=w779, "PRAMMS Error"=w778, "ROIWidth"=w774, "ROIHeight"=w773) -> ("Error"=w772:bool)  [unwired: 6 in]
              n562 = case shown="True" w772 {
                frame False {
                }
                frame True {
                  n563 = One Button Dialog(message="Une erreur est survenue lors de la configuration\nde la caméra de guidage.  Il se peut que certaines\nfonctionnalités ne soient pas disponibles.") -> ()  [unwired: 1 in, 1 out]
                }
              }
            }
            frame #2 {
              w782 = "emtAcknowlegment"
              n564 = local read "MessageType"() -> (w783:cluster{string[], u32[]})
              n565 = local read "Hexapod VRN"() -> (w797:refnum<visa-resource-name>)
              n566 = local read "PrAMS Error"() -> (w794:errorcluster)
              n567 = Type Cast(type=refnum<k5> refnum ("connection ID"), x=w797) -> (*(type *) &x=w799:refnum<k5>)
              n568 = local read "Signature"() -> (w790:u32)
              n569 = call-poly "SAOMM-Num2littleEndian.vi"("Number"="DefaultUAxisOffset") -> ("LiitleEndianedData"=w789:u8[])  [unwired: 14 in]
              n570 = call-poly "SAOMM-Num2littleEndian.vi"("Number"="DefaultVAxisOffset") -> ("LiitleEndianedData"=w788:u8[])  [unwired: 14 in]
              n571 = call "SendSET-NoListener.vi"("connection ID"=w799, "CommandArray"=w783, "ExpectedAnswer"=w782, "Signature"=w790, "Error IN"=w794, "Active SET"="emtSetUAxisOffset", "Value (little endianed byte array)"=w789) -> ("connection ID (dup)"=w792:refnum<k5>, "Succes"=→"SetUOffset":bool, "Error OUT"=w793:errorcluster)  [unwired: 6 in]
              n572 = call "SendSET-NoListener.vi"("connection ID"=w792, "CommandArray"=w783, "ExpectedAnswer"=w782, "Signature"=w790, "Error IN"=w793, "Active SET"="emtSetVAxisOffset", "Value (little endianed byte array)"=w788) -> ("Succes"=→"SetVOffset":bool, "Error OUT"=w791:errorcluster)  [unwired: 6 in, 1 out]
              n573 = local write "PrAMS Error"(w791) -> ()
            }
          }
        }
      }
    }
    frame #7 {
      # "- Ajustement des paramètres instrumentauux\n- Calcul des astrométries initiales\n- Initialisation des périphériques"
      n574 = case shown="True" w800 {
        frame False {
        }
        frame True {
          n575 = flat-sequence {
            tunnel: [TRUE] -> w804
            tunnel: w804 -> [w846]
            tunnel: [TRUE] -> w803
            tunnel: w803 -> [w888]
            tunnel: [TRUE] -> w802
            tunnel: w802 -> [w917]
            tunnel: [TRUE] -> w801
            frame #0 {
              # "Argh :("
              # "Fais la première commande #25 pour obtenir les infos du TCS, envoie la commande \"STOP\",\npuis force le TCS en mode \"EST\""
              n576 = control-ref of="TCS actif"() -> (w813:refnum<vi>)
              n577 = call "Fractional-Year.vi"() -> ("Fractional Year"=w810:dbl)  [unwired: 15 in]
              n578 = local read "TCS VRN"() -> (w814:refnum<visa-resource-name>)
              n579 = local read "dflt-EQX"() -> (w809:dbl)
              n580 = Build Array(w810) -> (w811:dbl[])
              n581 = call "EXCOM-CMD.vi"("VRN IN"=w814, "Bool Refnum"=w813, "Commande #"=22, "Args"=w811) -> ("VRN OUT"=w815:refnum<visa-resource-name>)  [unwired: 9 in, 2 out]
              n582 = call "EXCOM-25-EQ.vi"("VISA resource name"=w815, "Bool Refnum"=w813, "Display Equinox"=w809) -> ("HA"=w822:dbl, "RA"=w823:dbl, "Rotateur"=w807:dbl, "DEC"=w824:dbl, "Dome"=w830:dbl, "Epoque"=w825:dbl, "Focus"=w829:dbl, "VISA resource name dup"=w832:refnum<visa-resource-name>, "Masse d'air"=w826:dbl, "Temps Sidéral"=w827:dbl, "Temps Universel"=w828:dbl, "Année"=w831:dbl, "Error OUT"=w833:errorcluster)  [unwired: 2 in, 2 out]
              n583 = local write "RA Tel"(w823) -> ()
              n584 = local write "DEC Tel"(w824) -> ()
              n585 = local write "RotationTCS"(w807) -> ()
              n586 = local write "Angle Hor."(w822) -> ()
              n587 = local write "Dectmp"(w824) -> ()
              n588 = local write "Epoch Tel"(w825) -> ()
              n589 = local write "Coupole"(w830) -> ()
              n590 = local write "RAtmp"(w823) -> ()
              n591 = local write "Air Mass"(w826) -> ()
              n592 = local write "AnnéeRL"(w831) -> ()
              n593 = local write "LST"(w827) -> ()
              n594 = local write "UTC"(w828) -> ()
              n595 = local write "Foyer"(w829) -> ()
              n596 = call "SerialCommError.vi"("VISA IN"=w832, "error IN"=w833) -> ("VISA OUT"=w834:refnum<visa-resource-name>, "Error"=w817:bool, "error OUT"=w821:errorcluster)  [unwired: 11 in]
              n597 = Negate(x=w807) -> (-x=w806:dbl)
              n598 = expression code="x+90"(w806) -> (w805:dbl)
              n599 = case shown="True" w817 {
                tunnel: w827 -> [_ w838]
                tunnel: w825 -> [_ w837]
                tunnel: w824 -> [_ w836]
                tunnel: w823 -> [_ w835]
                frame False {
                }
                frame True {
                  n600 = call "Object_properties.vi"("Target RA"=w835, "Target DEC"=w836, "Target Epoch"=w837, "Sideral Time"=w838) -> ("NO RA"=w839:string, "NO DEC"=w840:string, "NO Epoch"=w842:dbl, "NO HA"=w841:dbl, "NO AM"=w843:dbl)  [unwired: 7 in]
                  n601 = local write "NO epoch"(w842) -> ()
                  n602 = local write "NO AM"(w843) -> ()
                  n603 = local write "NO HA"(w841) -> ()
                  n604 = local write "N.O. Déc."(w840) -> ()
                  n605 = local write "N.O. A.D."(w839) -> ()
                }
              }
              n606 = control-ref of="TCS actif"() -> (w816:refnum<vi>)
              n607 = local write "RotationEffective"(w805) -> ()
              n608 = call "EXCOM-CMD.vi"("VRN IN"=w834, "Bool Refnum"=w816, "Commande #"=13, "Error IN"=w821) -> ("VRN OUT"=w819:refnum<visa-resource-name>, "Error OUT"=w818:errorcluster)  [unwired: 9 in, 1 out]
              n609 = local write "TCS VRN"(w819) -> ()
              n610 = local write "TCS Error"(w818) -> ()
            }
            frame #1 {
              # "Demande l'instruments et synchronise Starry Night ..."
              # "Synchronise les coordonnées de StarryNight avec celle du télescope"
              n611 = local read "Instrument Actuel"() -> (w880:string)
              n612 = local read "SkipChoixInstr"() -> (w844:bool)
              n613 = local read "instruments.ini"() -> (w871:path)
              n614 = call "InstrChoice.vi"("Instrument IN"=w880, "SkipChoixInstr"=w844, "instruments.ini"=w871, "DisallowUndo"=TRUE) -> ("This VI's Path"=w865:path, "Instrument OUT"=w879:string, "FoV"=→"FOV":dbl, "foynom"=→"Foyer à 0°":i32, "atherm"=→"Ath_coef":dbl, "exclusion"=→"path_exclusion":path, "collim"=w848:path)  [unwired: 8 in, 1 out]
              "Instrument Actuel" <- w879
              n615 = Open VI Reference(vi path=w865) -> (vi reference=w855:refnum<vi>, error out=w854:errorcluster)  [unwired: 5 in]
              n616 = property class="VI"(reference=w855, error in=w854) -> (reference out=w859:refnum<vi>, error out=w858:errorcluster, "Front Panel.Open"=w857:bool)
              n617 = local read "Calib VRN"() -> (w869:refnum<visa-resource-name>)
              n618 = local read "Epoch Tel"() -> (w874:dbl)
              n619 = local read "RA Tel"() -> (w872:dbl)
              n620 = local read "DEC Tel"() -> (w873:dbl)
              n621 = Automation Open(Automation Refnum=refnum<k7> refnum ("ScopeSim._Telescope")) -> (Automation Refnum=w861:refnum<k7>)  [unwired: 3 in, 1 out]
              n622 = case shown="False" w857 {
                tunnel: w859 -> [_ w885]
                tunnel: w858 -> [w882 w884]
                tunnel: [w882 w883] -> w856
                frame False {
                }
                frame True {
                  n623 = invoke class="VI" method="FP.Close"(reference=w885, error in=w884) -> (error out=w883:errorcluster)  [unwired: 1 in, 2 out]
                }
              }
              n624 = local write "ActiveLUT"(w848) -> ()
              n625 = call "Controle_des_lampe.vi"("VISA resource name"=w869, "Status In"=bool[] [FALSE, FALSE, FALSE]) -> ("Status Out"=→"Status lamp":bool[])  [unwired: 2 out]
              n626 = Current VI's Menubar() -> (w878:refnum<k9>)
              n627 = call "Set_SN_Coords.vi"("Coords EPOCH"=w874, "input_DEC"=w873, "input_RA"=w872, "ScopeSim._Telescope"=w861) -> ("precessed_DEC"=w863:dbl, "precessed_RA"=w864:dbl)  [unwired: 6 in]
              n628 = global write "Globals.vi" "ScopeSim._Telescope"(w861) -> ()
              n629 = local write "VI Reference Error"(w856) -> ()
              n630 = Set Menu Item Info(6:TRUE ("coché"), 7:w879, 11:w878) -> (0:w866:errorcluster)  [unwired: 4 in, 1 out]
              n631 = local write "Dectmp"(w863) -> ()
              n632 = local write "RAtmp"(w864) -> ()
              n633 = call "SAOMM-XML2LUT.vi"("Path"=w848) -> ("NominalPositions"=w847:dbl[])  [unwired: 13 in, 1 out]
              n634 = local write "Menu Error"(w866) -> ()
              n635 = Index Array(array=w847) -> (element #3=w853:dbl, element #4=w852:dbl, element #5=w851:dbl, element #6=w850:dbl, element #7=w849:dbl)  [unwired: 7 in, 2 out]
              n636 = local write "Nominal Y"(w852) -> ()
              n637 = local write "Nominal X"(w853) -> ()
              n638 = local write "Nominal Z"(w851) -> ()
              n639 = local write "Nominal V"(w849) -> ()
              n640 = local write "Nominal U"(w850) -> ()
              "Initialisation TCS" <- w846
            }
            frame #2 {
              # "Initialisation des tables de guidages et de la connexion au simulateur de TELESCOPE\n\n possiblement qu'il faudra ajouter l'origine automatique des systèmes SAOMM"
              n641 = local read "Table VRN"() -> (w891:refnum<visa-resource-name>)
              n642 = local read "vitesse lente"() -> (w895:dbl)
              n643 = local read "accelleration"() -> (w893:dbl)
              n644 = control-ref of="Table actif"() -> (w892:refnum<vi>)
              n645 = local read "vitesse rapide"() -> (w894:dbl)
              n646 = local read "ActiveStages"() -> (w886:string[])
              "ActiveStages" <- w886
              n647 = for {
                tunnel: w886 -> [w902] mode=indexing
                tunnel: w895 -> [w903]
                tunnel: w894 -> [w904]
                tunnel: w893 -> [w905]
                tunnel: w892 -> [w906]
                tunnel: w891 -> [w909]
                tunnel: [w908] -> w890
                tunnel: [w907] -> w889
                n648 = call "Newmark-SetSpeed.vi"("Table VRN"=w909, "StageTAG"=w902, "Bool Refnum"=w906, "Vitesse Lente"=w903, "Vitesse Rapide"=w904, "Accélération"=w905) -> ("Table VRN OUT"=w908:refnum<visa-resource-name>, "Error OUT"=w907:errorcluster)  [unwired: 7 in, 1 out]
              }
              n649 = property on="Origine" class="Bool (strict)"("Blinking"=TRUE) -> ()  [unwired: 2 in, 2 out]
              n650 = call "Newmark-QueryPosition.vi"("Table VRN IN"=w890, "Bool Refnum"=w892, "Error IN"=w889) -> ("X Axis"=w898:dbl, "Y Axis"=w897:dbl, "Table VRN OUT"=w900:refnum<visa-resource-name>, "Z Axis"=w896:dbl, "Error OUT"=w899:errorcluster)  [unwired: 5 in, 3 out]
              n651 = local write "Table VRN"(w900) -> ()
              n652 = local write "Table Error"(w899) -> ()
              n653 = local write "Position X"(w898) -> ()
              n654 = local write "Position Y"(w897) -> ()
              n655 = local write "Position Z"(w896) -> ()
              "Choix de l'insturment" <- w888
            }
            frame #3 {
              w910 = 0.0
              w931 = u16 0 items=["Square", "Circle"] ("Ring")
              # "Invert X"
              # "Époque DSS et USNO"
              # "Seul le champ est approximé, dans un avenir lointain\non pourra tenir compte de la distorsion en ajoutant\nla structure de distortion décrite dans Calabretta et al 2004"
              n656 = local read "arcsec/pulse"() -> (w934:dbl)
              n657 = local read "CentreTel X"() -> (w940:dbl)
              n658 = local read "CentreTel Y"() -> (w941:dbl)
              n659 = local read "Reference X"() -> (w939:dbl)
              n660 = local read "Reference Y"() -> (w938:dbl)
              n661 = local read "RA Tel"() -> (w936:dbl)
              n662 = local read "DEC Tel"() -> (w935:dbl)
              n663 = local read "MirVig"() -> (w913:dbl)
              n664 = local read "Miroir"() -> (w912:dbl)
              n665 = local read "RotationEffective"() -> (w915:dbl)
              n666 = local read "Représentation"() -> (w920:dbl)
              n667 = local read "Epoch Tel"() -> (w926:dbl)
              n668 = local read "FOV"() -> (w930:dbl)
              n669 = Bundle("MirVig"=w913, w910, w910, "Miroir"=w912) -> (w911:cluster{"MirVig":dbl, dbl, dbl, "Miroir":dbl})  [unwired: 1 in]
              n670 = call "Set_field_astrometry.vi"("Cen x (pas)"=w940, "effective rotation (°)"=w915, "scale (\"/pas)"=w934, "NaxisMax"=500000, "Cen y (pas)"=w941, "Use Center?"=FALSE, "Ref x (pas)"=w939, "Ref y (pas)"=w938, "RA (HH:MM:SS.S)"=w936, "DEC(DD:MM:SS)"=w935, "Inversion Cluster"=T20 {"Invert Angle"=FALSE, "Invert X"=TRUE, "Invert Y"=FALSE}) -> ("Field Astrometry"=w927:T4, "Table Astrometry"=w928:T4)  [unwired: 3 in]
              "FieldAstrom" <- w927
              n671 = call "draw_field.vi"("Field_Astrometry"=w927, "FOV"=w930, "Ring"=w931, "Table_Astrometry"=w928, "Ues Constant Size ?"=TRUE, "margin/size"=w920, "MirrorAvatar"=w911) -> ("TableXYPos"=w921:cluster{dbl[], dbl[]}[], "X Scale.Range"=w932:T26, "ImgDEC"=w914:dbl, "ImgRA"=w924:dbl, "Y Scale.Range"=w933:T26)  [unwired: 4 in]
              n672 = local write "TableAstrom"(w928) -> ()
              n673 = call "precess.vi"("Eq2"=2000.0, "Eq1"=w926, "DEC 1"=w914, "RA 1"=w924) -> ("DEC 2"=w922:dbl, "RA 2"=w923:dbl)
              n674 = local write "DEC-Champ"(w922) -> ()
              n675 = property on="TableXYPos" class="XYGraph (strict)"("Value"=w921, "XScale.Range"=w932, "YScale.Range"=w933) -> ()  [unwired: 2 in, 2 out]
              n676 = local write "RA-Champ"(w923) -> ()
              "Vitesse des tables" <- w917
            }
          }
          "Astrométries" <- w801
        }
      }
    }
    frame #8 {
      # "Boucle principale du programme"
      n677 = case shown="True" w943 {
        frame False {
        }
        frame True {
          (unwired) TRUE
          # "Hexapode Listener"
          n678 = while {
            tunnel: ["Quit"] -> w956
            stop <- "Quit" stop-if-true
            # "Structure de gestion des événements utilisateurs"
            n679 = event shown="[24] \"ModifFoyer\": Value Change" {
              selector: _ -> [_ _ _ _ _ _ _ _ _ _ _ _ _ _ _ _ _ _ _ _ _ _ _ _ _ _ _ _ _ _ _ _ _ _ _ _ _ _ _ _ _ _ _ _ _ _ _ _ _ _ _ _ _ _ _ _ _ _ _ _ _ _ _ _ _ _ _]
              dyn-events: _ -> [_ _ _ _ _ _ _ _ _ _ _ _ _ _ _ _ _ _ _ _ _ _ _ _ _ _ _ _ _ _ _ _ _ _ _ _ _ _ _ _ _ _ _ _ _ _ _ _ _ _ _ _ _ _ _ _ _ _ _ _ _ _ _ _ _ _ _]
              timeout: 250 -> [_ _ _ _ _ _ _ _ _ _ _ _ _ _ _ _ _ _ _ _ _ _ _ _ _ _ _ _ _ _ _ _ _ _ _ _ _ _ _ _ _ _ _ _ _ _ _ _ _ _ _ _ _ _ _ _ _ _ _ _ _ _ _ _ _ _ _]
              event Timeout {
                w3946 = FALSE
                # "S'il y a un problème avec MC-BonOMM, regarder ici ;)"
                # "Test pour les boutons de Jog ..."
                n680 = event-data() -> ()  [unwired: 1 in, 1 out]
                n681 = local write "Annulation en cours"(FALSE) -> ()
                n682 = disable-structure shown="Enabled" {
                  frame Disabled {
                    n683 = local read "MC-BonOMM VRN"() -> (w3948:refnum<visa-resource-name>)
                    n684 = property class="Instr"(reference=w3948) -> (reference out=w3949:refnum<visa-resource-name>, "Serial Settings:Number of Bytes at Serial Port"=w3950:u32)  [unwired: 1 in, 1 out]
                    n685 = VISA Read(VISA resource name=w3949, byte count=w3950) -> ()  [unwired: 1 in, 4 out]
                  }
                  frame Enabled {
                  }
                }
                n686 = local write "go Nord"(w3946) -> ()
                n687 = local write "go Ouest"(w3946) -> ()
                n688 = local write "go Est"(w3946) -> ()
                n689 = local write "go Sud"(w3946) -> ()
                n690 = local write "enfoncé"(w3946) -> ()
              }
              event Menu Selection (User) {
                n691 = event-data() -> ("MenuRef"=w3951:refnum<k9>, "ItemTag"=w3953:string, "ItemPath"=w3954:string)  [unwired: 1 in, 3 out]
                n692 = Concatenate Strings(":" ("search string/char (-)"), w3953) -> (w3955:string)
                n693 = Search/Split String(string=w3954, search string/char (-)=w3955) -> (substring before match=w3952:string)  [unwired: 1 in, 2 out]
                n694 = case shown="\"main_Télescope\"" w3952 {
                  tunnel: w3953 -> [_ w3957 w4274 w4305 w4391 w4466 w4560 w4654 w4715]
                  tunnel: w3951 -> [_ _ _ _ _ _ w4559 _ _]
                  frame Default {
                  }
                  frame "main_Communications" {
                    # "Gestion des éléments du menu \"communications\"\n(fermeture de la connexion, puis redémarrage)"
                    n695 = case shown="\"com_MC-BonOMM\"" w3957 {
                      frame Default {
                        (unwired) FALSE ("Boolean")
                      }
                      frame "com_Telescope Control System" {
                        n696 = flat-sequence {
                          frame #0 {
                            w3971 = "communications" ("name or relative path")
                            n697 = control-ref of="TCS actif"() -> (w3960:refnum<vi>)
                            n698 = local read "TCS VRN"() -> (w3965:refnum<visa-resource-name>)
                            n699 = call "EXCOM-25-EQ.vi"("VISA resource name"=w3965, "Bool Refnum"=w3960) -> ("VISA resource name dup"=w3963:refnum<visa-resource-name>, "Error OUT"=w3964:errorcluster)  [unwired: 3 in, 13 out]
